vi "NanotecSMCPDDriver.revision query.vi"(0 "VISA resource name":refnum<visa-resource-name>, 1 "contollerID":i32=-1, 5 "error in (no error)":errorcluster) -> (14 "VISA resource name out":refnum<visa-resource-name>, 15 "contollerID out":i32=-1, 16 "Instrument Driver Revision":string, 17 "Instrument Firmware Revision":string, 19 "error out":errorcluster)   [LabVIEW 2014, in "NanotecSMCPDDriver.lvlib"]
doc: "Queries the current instrument firmware revision and instrument driver revision.\n\nRefer to the Readme file for detailed driver information including modification history."
uses:
  NanotecSMCPDDriver.lvlib
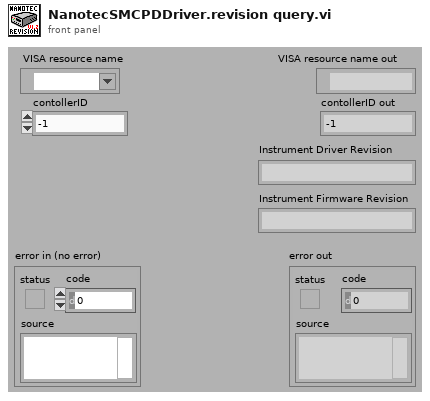
[diagram p1: front panel]
types:
  T1 = cluster{"Major":u16, "Minor":u16, "Fix":u16, "Build":u16}
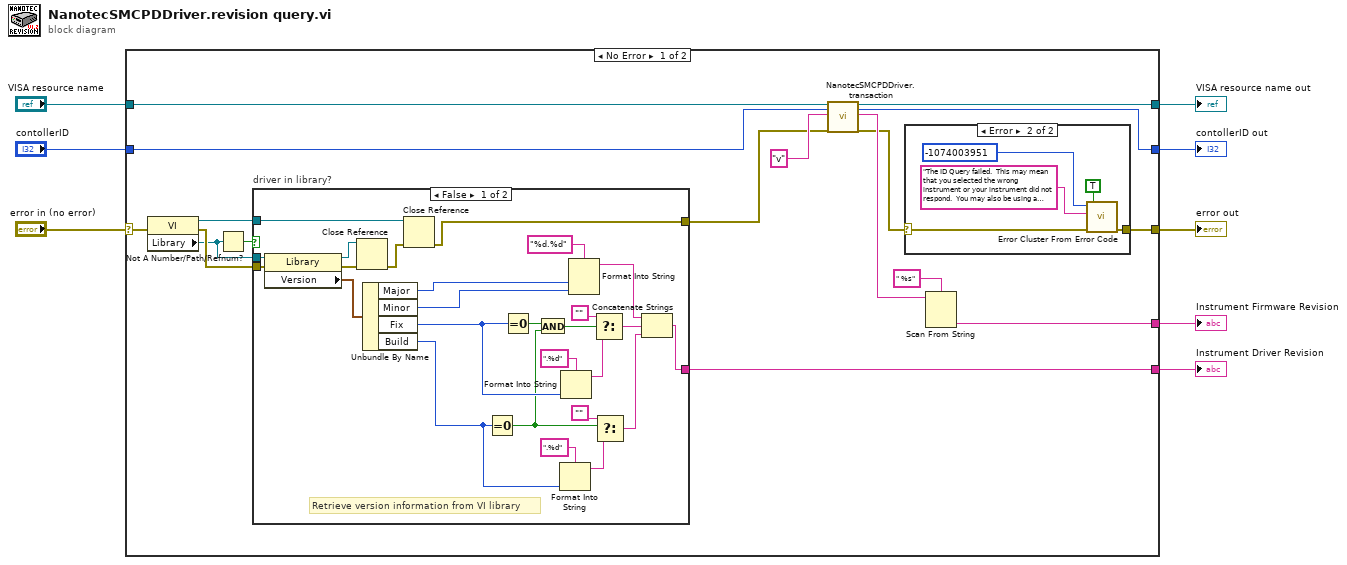
[diagram p0: block diagram]
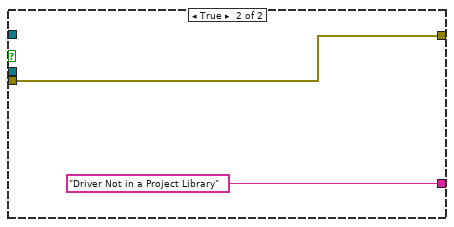
[diagram p3: hidden frame]
diagram:
  n1 = case shown="No Error" "error in (no error)" {
    selector: "error in (no error)" -> [w13 w60]
    tunnel: [w11 w62] -> w8
    tunnel: [w9 w60] -> w7
    tunnel: "VISA resource name" -> [w21 w62]
    tunnel: "contollerID" -> [w18 w61]
    tunnel: [w17 w61] -> w4
    tunnel: [w14 _] -> w3
    tunnel: [w12 _] -> w1
    frame No Error {
      n2 = property on="Property Node" class="VI"(error in=w13) -> (reference out=w25:refnum<vi>, error out=w24:errorcluster, "Library"=w23:refnum<vi>)  [unwired: 1 in]
      n3 = Not A Number/Path/Refnum?(number/path/refnum=w23) -> (NaN/Path/Refnum?=w22:bool)
      n4 = case "driver in library?" shown="False" w22 {
        tunnel: w25 -> [w54 _]
        tunnel: w24 -> [w39 w59]
        tunnel: [w34 w59] -> w19
        tunnel: [w33 "Driver Not in a Project Library"] -> w12
        tunnel: w23 -> [w32 _]
        frame False {
          # "Retrieve version information from VI library"
          n5 = property on="Property Node" class="Library"(reference=w32, error in=w39) -> (reference out=w56:refnum<vi>, error out=w57:errorcluster, "Version"=w53:T1)
          n6 = Close Reference(reference=w56, error in (no error)=w57) -> (error out=w55:errorcluster)
          n7 = Unbundle By Name(w53) -> ("Major"=w42:u16, "Minor"=w41:u16, "Fix"=w38:u16, "Build"=w40:u16)
          n8 = Close Reference(reference=w54, error in (no error)=w55) -> (error out=w34:errorcluster)
          n9 = Equal To 0?(x=w40) -> (x = 0?=w36:bool)
          n10 = Equal To 0?(x=w38) -> (x = 0?=w37:bool)
          n11 = And(x=w37, y=w36) -> (x .and. y?=w35:bool)
          n12 = Format Into String(format string=".%d", w40) -> (resulting string=w46:string)  [unwired: 2 in, 1 out]
          n13 = Format Into String(format string=".%d", w38) -> (resulting string=w50:string)  [unwired: 2 in, 1 out]
          n14 = Format Into String(format string="%d.%d", w42, w41) -> (resulting string=w48:string)  [unwired: 2 in, 1 out]
          n15 = Select(t="" ("Empty String Constant"), s=w35, f=w50) -> (s? t:f=w47:string)
          n16 = Select(t="" ("Empty String Constant"), s=w36, f=w46) -> (s? t:f=w43:string)
          n17 = Concatenate Strings(w48, w47, w43) -> (w33:string)
        }
        frame True {
        }
      }
      n18 = call "NanotecSMCPDDriver.transaction.vi"("VISAresource"=w21, "contollerID"=w18, "commandString"="v", "error in (no error)"=w19) -> ("VISAresource out"=w11:refnum<visa-resource-name>, "contollerID out"=w17:i32, "response"=w16:string, "error out"=w10:errorcluster)  [unwired: 10 in, 2 out]
      n19 = case shown="Error" w10 {
        selector: w10 -> [w26 w28]
        tunnel: [w26 w27] -> w9
        frame No Error {
        }
        frame Error {
          n20 = call <vilib>:"Error Cluster From Error Code.vi"("show call chain? (False)"=TRUE, "error in (no error)"=w28, "error message (\"\")"="The ID Query failed.  This may mean that you selected the wrong instrument or your instrument did not respond.  You may also be using a model that is not officially supported by this driver.  If you are sure that you have selected the correct instrument and it is responding, try disabling the ID Query." ("Source (VI Name)"), "error code (0)"=-1074003951 ("Code")) -> ("error out"=w27:errorcluster)  [unwired: 5 in]
        }
      }
      n21 = Scan From String(format string=" %s", input string=w16) -> (output 1=w14:string)  [unwired: 3 in, 3 out]
    }
    frame Error {
    }
  }
  "Instrument Firmware Revision" <- w3
  "VISA resource name out" <- w8
  "error out" <- w7
  "contollerID out" <- w4
  "Instrument Driver Revision" <- w1
